vi "BuildMenu3.vi"(8 "Click Type":T1, 9 "Point":T2, 10 "XRef":refnum<vi>, 11 "State In":T10) -> (1 "Show Standard Items? (Popup click only)":bool=TRUE, 2 "Menu Specification":T4)   [LabVIEW 2012, in "Minimum Array Size.xnode"]
doc: "If you are seeing this VI, you have asked the XNode Manager for an ability is not defined in the Blank XNode. If you are trying new abilities, go ahead. If not, please inform of this error."
uses:
  Minimum Array Size.xnode
  State.ctl
  <vilib>/XNodeSupport/XNodeMenuSpecs3.ctl
  <vilib>/XNodeSupport/XNodeMenuSpec3.ctl
  <vilib>/XNodeSupport/XNodeString.ctl
  <vilib>/XNodeSupport/XNodeBool.ctl
  <vilib>/XNodeSupport/XNodeStandardHelpInfo.ctl
  <vilib>/XNodeSupport/XNodePath.ctl
  <vilib>/XNodeSupport/XNodePoint.ctl
  <vilib>/XNodeSupport/XNodeInt.ctl
  <vilib>/XNodeSupport/XNodeClickTypes.ctl
  <vilib>/XNodeSupport/NI_XNodeSupport.lvlib
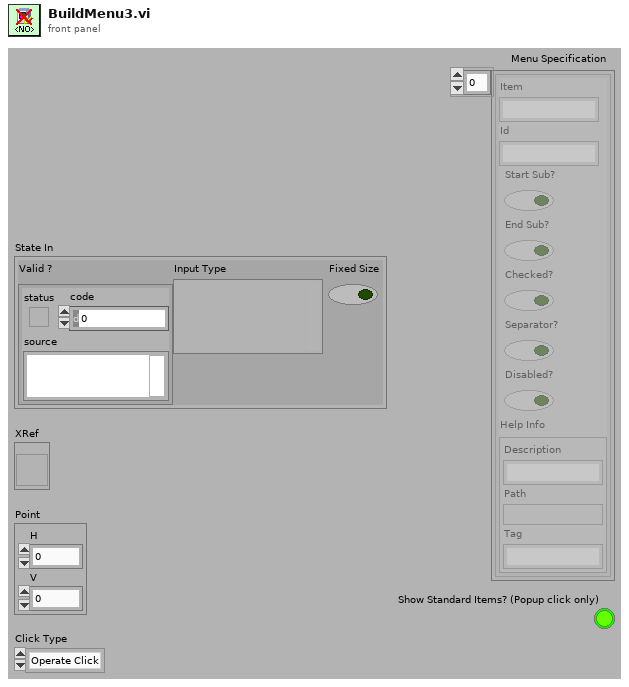
[diagram p1: front panel]
types:
  T1 = typedef "NI_XNodeSupport.lvlib/XNodeClickTypes.ctl" = enum32{"Operate Click", "Popup Click"}
  T2 = typedef "NI_XNodeSupport.lvlib/XNodePoint.ctl" = cluster{"H":T3, "V":T3}
  T3 = typedef "NI_XNodeSupport.lvlib/XNodeInt.ctl" = i32
  T4 = typedef "NI_XNodeSupport.lvlib/XNodeMenuSpecs3.ctl" = T5[]
  T5 = typedef "NI_XNodeSupport.lvlib/XNodeMenuSpec3.ctl" = cluster{"Item":T6, "Id":T6, "Start Sub?":T7, "End Sub?":T7, "Checked?":T7, "Separator?":T7, "Disabled?":T7, "Help Info":T8}
  T6 = typedef "NI_XNodeSupport.lvlib/XNodeString.ctl" = string
  T7 = typedef "NI_XNodeSupport.lvlib/XNodeBool.ctl" = bool
  T8 = typedef "NI_XNodeSupport.lvlib/XNodeStandardHelpInfo.ctl" = cluster{"Description":T6, "Path":T9, "Tag":T6}
  T9 = typedef "NI_XNodeSupport.lvlib/XNodePath.ctl" = path
  T10 = typedef "Minimum Array Size.xnode/State.ctl" = cluster{"Valid ?":errorcluster, "Input Type":variant, "Fixed Size":bool}
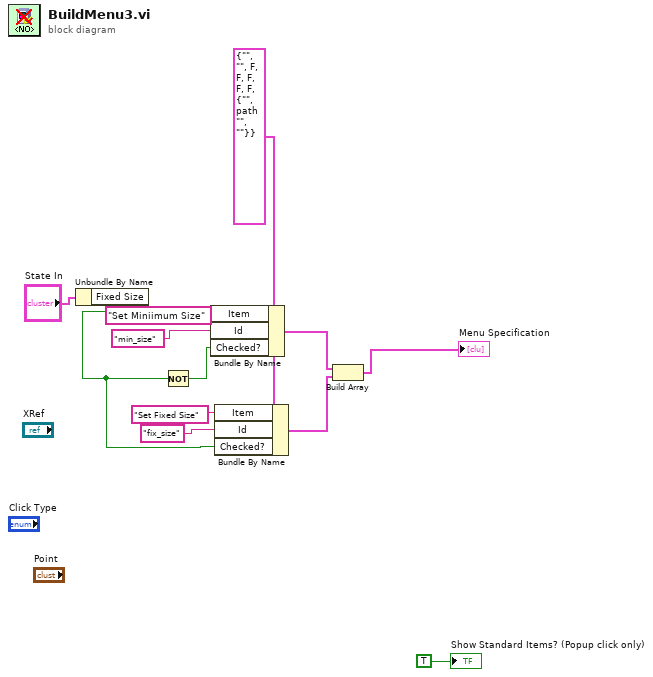
[diagram p0: block diagram]
diagram:
  w8 = T5 {"Item"="", "Id"="", "Start Sub?"=FALSE, "End Sub?"=FALSE, "Checked?"=FALSE, "Separator?"=FALSE, "Disabled?"=FALSE, "Help Info"={"Description"="", "Path"=path "", "Tag"=""}} ("Menu Item 3")
  n1 = Unbundle By Name("State In") -> ("Fixed Size"=w6:bool)
  n2 = Not(x=w6) -> (.not. x?=w7:bool)
  n3 = Bundle By Name(cluster=w8, "Item"=T6 "Set Miniimum Size", "Id"=T6 "min_size", "Checked?"=w7) -> (w3:T5)
  n4 = Bundle By Name(cluster=w8, "Item"=T6 "Set Fixed Size", "Id"=T6 "fix_size", "Checked?"=w6) -> (w2:T5)
  n5 = Build Array(w3, w2) -> (→"Menu Specification":T5[])
  "Show Standard Items? (Popup click only)" <- TRUE ("Show Standard Items? (Popup click only)")
